vi "Get SMO RC Type.vi"(8 "error in (no error)":errorcluster, 11 "Inst.Attocube-3DRInstrument in":refnum<class "Inst.Attocube-3DR.lvclass">) -> (0 "error out":errorcluster, 2 "RemoteControl":refnum<class "RemoteControl.lvclass">, 3 "Inst.Attocube-3DRInstrument out":refnum<class "Inst.Attocube-3DR.lvclass">)   [LabVIEW 2019, in "Inst.Attocube-3DR.lvclass"]
uses:
  Inst.Attocube-3DR.lvclass
  <userlib>/LevyLab/Instrument Framework/Instrument/Instrument.lvclass
  <userlib>/LevyLab/RemoteControl/RemoteControl/RemoteControl.lvclass
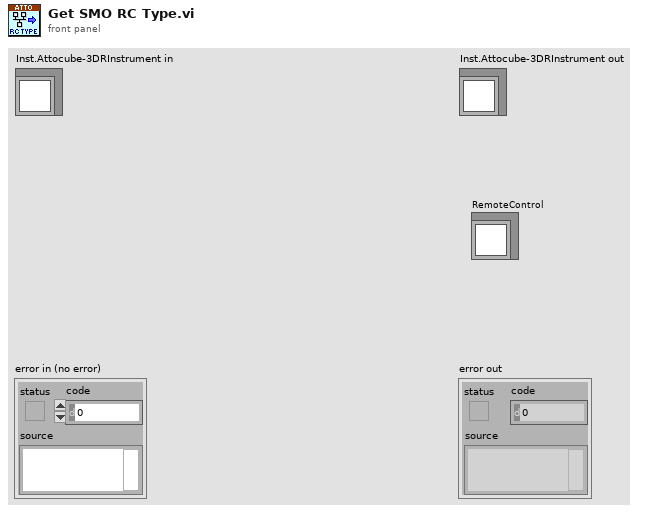
[diagram p1: front panel]
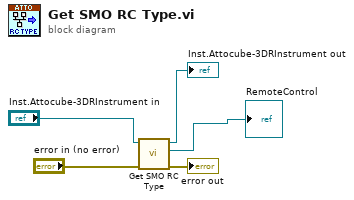
[diagram p0: block diagram]
diagram:
  n1 = call-parent "Get SMO RC Type.vi"("error in (no error)"="error in (no error)", "Instrument in"="Inst.Attocube-3DRInstrument in") -> ("error out"=→"error out":errorcluster, "RemoteControl"=→"RemoteControl":refnum<class "RemoteControl.lvclass">, "Instrument out"=→"Inst.Attocube-3DRInstrument out":refnum<class "Inst.Attocube-3DR.lvclass">)  [unwired: 7 in]
